vi "Level Set S&THx.vi"() -> ()   [LabVIEW 2017]
panel:
  out "Level Set":dbl
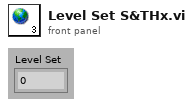
[diagram p1: front panel]
diagram:
